vi "Median Filter.vi"(7 "Initial Value":dbl, 11 "Variable":dbl) -> (3 "Filtered Value":dbl format="%0.2f")   [LabVIEW 2013]
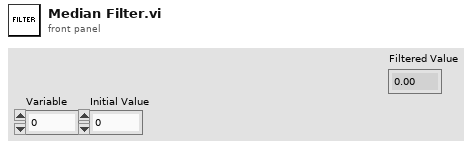
[diagram p1: front panel]
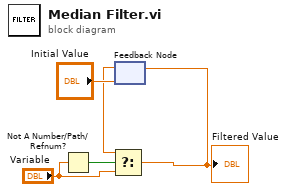
[diagram p0: block diagram]
diagram:
  n1 = Not A Number/Path/Refnum?(number/path/refnum="Variable") -> (NaN/Path/Refnum?=w2:bool)
  n2 = feedback #1("Initial Value") -> (w3:dbl)
  n3 = Select(t=w3, s=w2, f="Variable") -> (s? t:f=w1:dbl)
  "Filtered Value" <- w1
  n4 = feedback-in #1(w1) -> ()
